vi "MGCC_FntStaMach_Closeall.vi"() -> ()   [LabVIEW 2016]
uses:
  Communication/Global communication output.vi
  Communication/Global communication.vi
panel:
  in  "Relay":bool[](array[boolean])=[FALSE, FALSE, FALSE, FALSE, FALSE, FALSE, FALSE, FALSE]
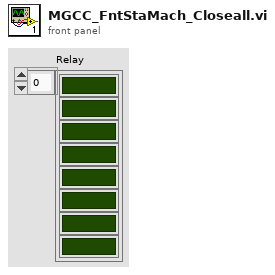
[diagram p1: front panel]
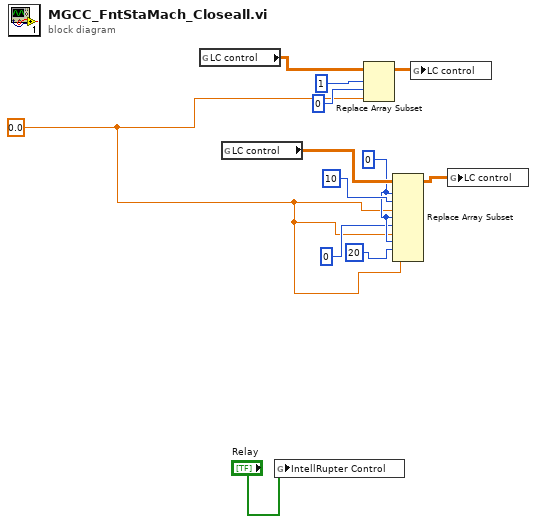
[diagram p0: block diagram]
diagram:
  w2 = 0.0 ("new element/subarray")
  w5 = 0 ("index")
  n1 = global read "Global communication.vi" "LC control"() -> (w11:dbl[][])
  n2 = global read "Global communication.vi" "LC control"() -> (w9:dbl[][])
  n3 = global write "Global communication output.vi" "IntellRupter Control"("Relay") -> ()
  n4 = Replace Array Subset(array=w11, new element=w2, index (row)=1 ("index"), index (col)=0 ("index")) -> (w10:dbl[][])
  n5 = Replace Array Subset(array=w9, new element #1=w2, index (row) #1=w5, index (col) #1=10 ("index"), new element #2=w2, index (row) #2=w5, index (col) #2=0 ("index"), new element #3=w2, index (row) #3=w5, index (col) #3=20 ("index")) -> (w8:dbl[][])
  n6 = global write "Global communication.vi" "LC control"(w10) -> ()
  n7 = global write "Global communication.vi" "LC control"(w8) -> ()
